vi "simulation data VI.vi"(1 "Boolean":bool, 2 "Volume Dispensed":string, 3 "Solution":string, 4 "Time Stamp 2":timestamp) -> (0 "Cluster":T1 {"Time Stamp" format="%<%.3X>T"})   [LabVIEW 2020]
uses:
  Controls/SImulation Data.ctl
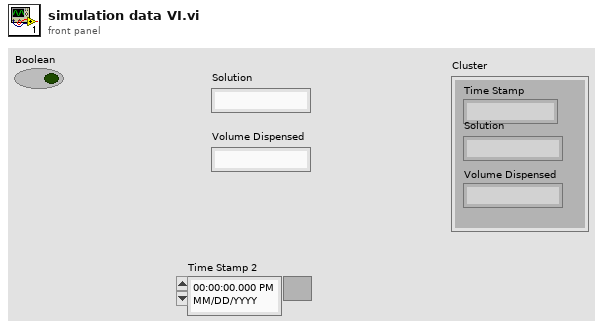
[diagram p1: front panel]
types:
  T1 = typedef "SImulation Data.ctl" = cluster{"Time Stamp":timestamp, "Solution":string, "Volume Dispensed":string}
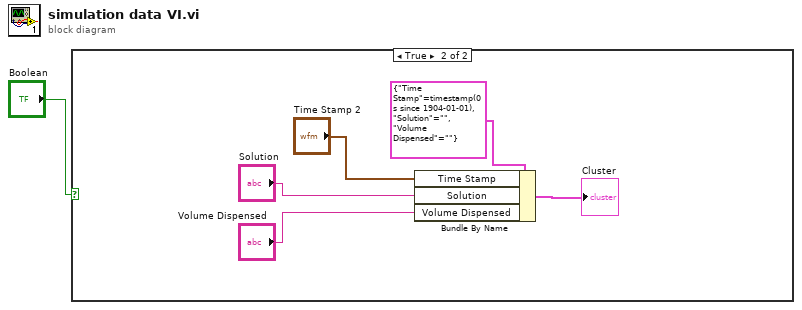
[diagram p0: block diagram]
diagram:
  n1 = case shown="True" "Boolean" {
    frame False {
    }
    frame True {
      n2 = Bundle By Name(cluster=T1 {"Time Stamp"=timestamp(0 s since 1904-01-01), "Solution"="", "Volume Dispensed"=""} ("Cluster"), "Time Stamp"="Time Stamp 2", "Solution"="Solution", "Volume Dispensed"="Volume Dispensed") -> (→"Cluster":T1)
    }
  }
